vi "Set_Traverse_Position.vi"(3 "Last Part of Move?":bool=TRUE, 4 "Currently on Point":i32=11, 5 "Simulate/Run":T3, 6 "Traverse line":T4 {"Carrier_2 Q (l/min)" format="%#.2f"; "Row Duration (mins)" format="%#.1f"; "Row No" min=0; "Trace Gas Concentration (%)" min=0.0 format="%#_4f"; "Carrier_1 Q (l/min)" format="%#.4f"; "Start X" format="%#.2f"; "Start Y" format="%#.2f"; "Start Z" format="%#.2f"; "End X" format="%#.2f"; "End Y" format="%#.2f"; "End Z" format="%#.2f"; "Tunnel Speed" format="%#.2f"; "Averaging time (mins)" min=0.0 format="%#.2f"}) -> (0 "Status Cluster":T1)   [LabVIEW 2021]
uses:
  Traverse_cluster.ctl
  Spacing.ctl
  Controls/Multi_run_mode.ctl
  Controls/User_Specific_mode.ctl
  Status_Cluster.ctl
  Multi_Run_Status.ctl
  Controls/Home.ctl
  Globals/Extra_Commands_Global.vi
  Globals/Dynamic_call_global.ph.vi
  Globals/Constants_global.vi
panel:
  # "X           Y          Z"
  # "Start"
  # "End"
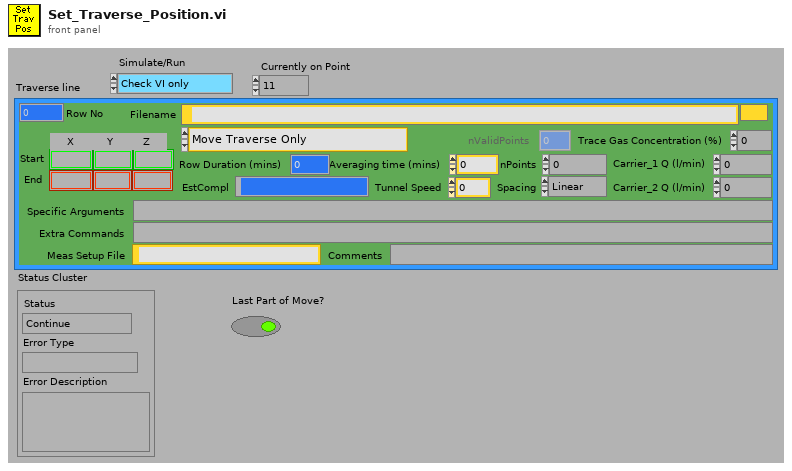
[diagram p1: front panel]
types:
  T1 = typedef "Status_Cluster.ctl" = cluster{"Status":T2, "Error Type":string, "Error Description":string}
  T2 = typedef "Multi_Run_Status.ctl" = enum16{"Continue", "Continue with Error", "Jump to Next Point", "Jump to Next Row", "Jump To Fall Back", "Terminate Run"}
  T3 = typedef "User_Specific_mode.ctl" = enum16{"Check VI only", "Run VI"}
  T4 = typedef "Traverse_cluster.ctl" = cluster{"Start X":sgl, "Start Y":sgl, "Start Z":sgl, "End X":sgl, "End Y":sgl, "End Z":sgl, "nPoints":i32, "Spacing":T5, "Filename":path, "Tunnel Speed":dbl, "Averaging time (mins)":dbl, "Extra Commands":string, "Carrier_1 Q (l/min)":dbl, "Carrier_2 Q (l/min)":dbl, "Trace Gas Concentration (%)":dbl, "Specific Arguments":string, "Comments":string, "Row No":i32, "Row Type Selector":T6, "EstCompl":string, "Row Duration (mins)":dbl, "nValidPoints":i32, "Meas Setup File":string}
  T5 = typedef "Spacing.ctl" = enum16{"Linear", "Log", "Gauss", "Specified", "N/A"}
  T6 = typedef "Multi_run_mode.ctl" = enum16{"Move Traverse Only", "Set Tunnel Speed Only", "Set Source Only", "Set Measurement Conditions", "Single Measurement", "Vertical Profile", "Lateral Profile", "Longitudinal Profile", "Multi-Axis Profile", "Explore Volume", "Auto Calibrate", "Meas Fast FID Bkgnd", "Check Beam Power", "Scanning Valve Measurement", "Run VI Named:", "Set ADAM Ch", "Wait (minutes)", "Send Message", "Synchronize With:", "Fall Back to this Row", "Turn Off Row Repeating", "Traverse 3D Volume", "Blank Row", "Jump to Fall Back Row"}
  T7 = typedef "Home.ctl" = enum16{"Don't Home", "Home  +X", "Home  -X", "Home  +Y", "Home  -Y", "Home  +Z", "Home  -Z"}
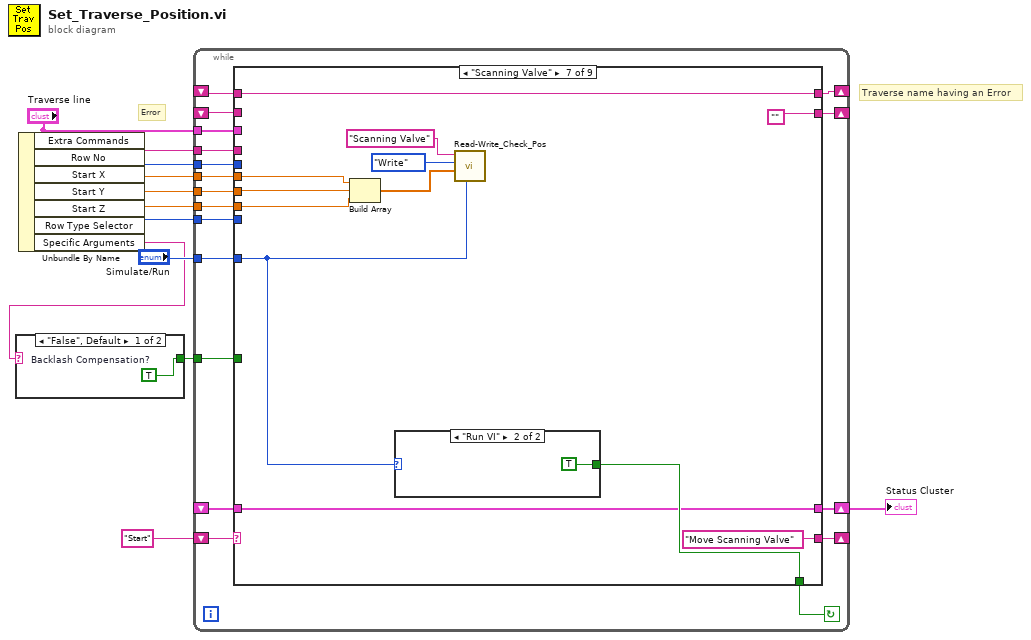
[diagram p0: block diagram]
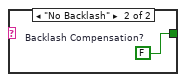
[diagram p2: hidden frame]
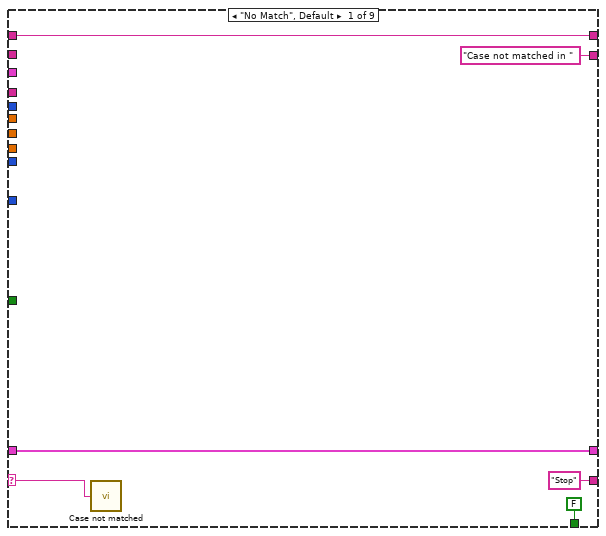
[diagram p3: hidden frame]
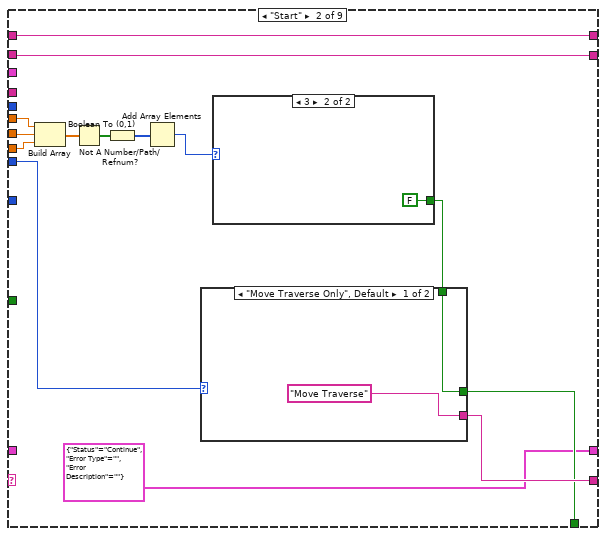
[diagram p4: hidden frame]
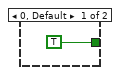
[diagram p5: hidden frame]
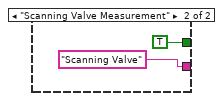
[diagram p6: hidden frame]
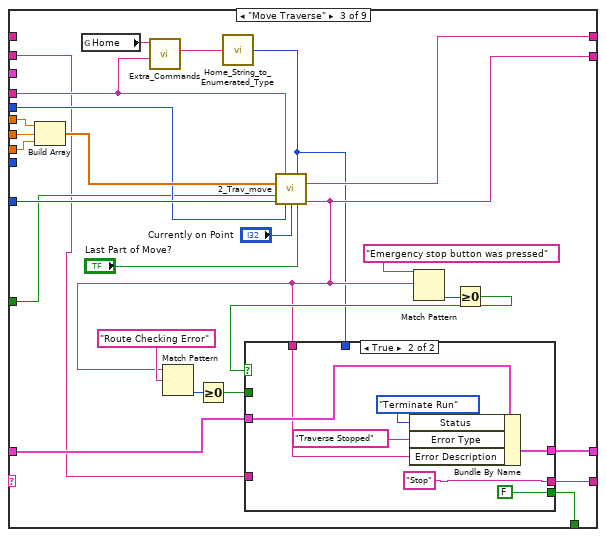
[diagram p7: hidden frame]
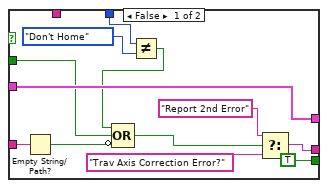
[diagram p8: hidden frame]
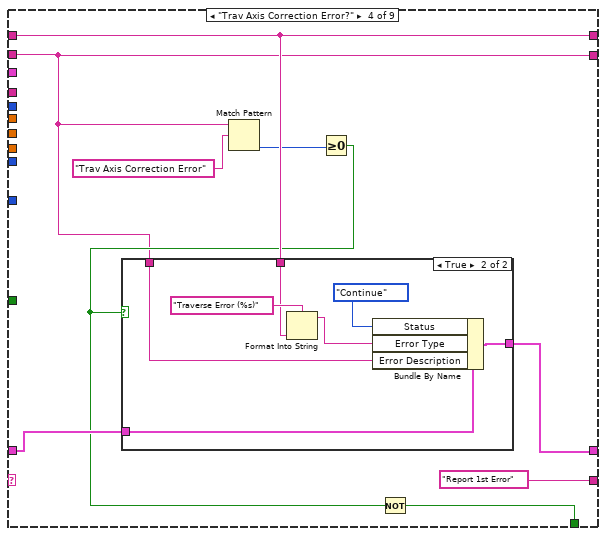
[diagram p9: hidden frame]
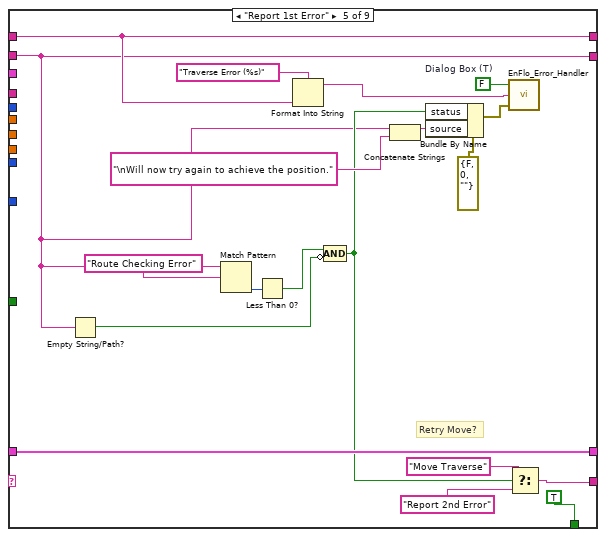
[diagram p11: hidden frame]
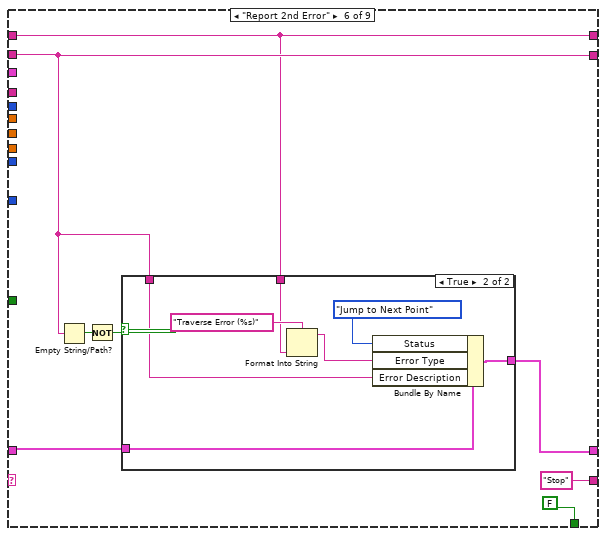
[diagram p12: hidden frame]
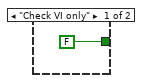
[diagram p14: hidden frame]
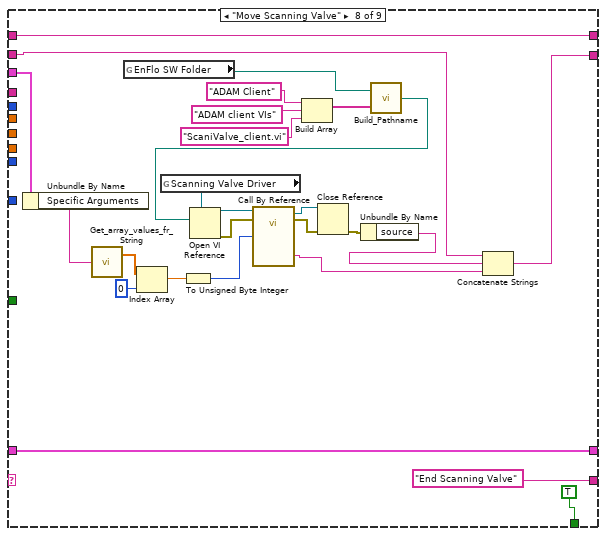
[diagram p15: hidden frame]
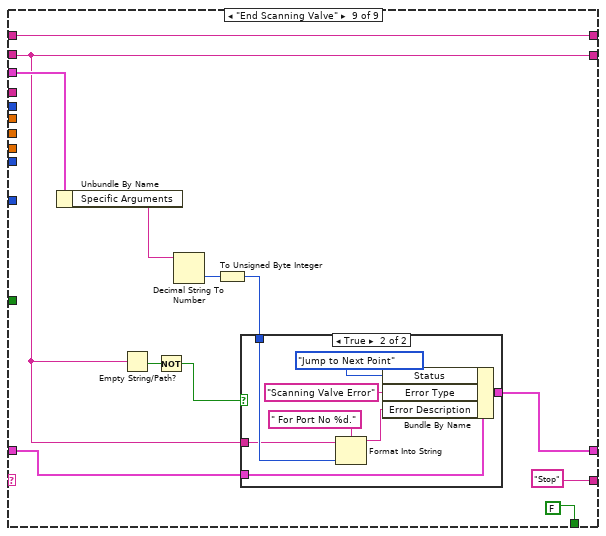
[diagram p16: hidden frame]
diagram:
  # "Traverse name having an Error"
  # "Error"
  n1 = Unbundle By Name("Traverse line") -> ("Extra Commands"=w11:string, "Row No"=w10:i32, "Start X"=w8:sgl, "Start Y"=w12:sgl, "Start Z"=w7:sgl, "Row Type Selector"=w9:T6, "Specific Arguments"=w3:string)
  n2 = case shown="\"False\", Default" w3 {
    tunnel: [w13 w14] -> w2
    frame "False", Default {
      w13 = TRUE  # Backlash Compensation?
    }
    frame "No Backlash" {
      w14 = FALSE  # Backlash Compensation?
    }
  }
  n3 = while {
    shift-left: _ -> [w19]
    shift-right: [w20] -> _
    shift-left: _ -> [w21]
    shift-right: [w22] -> w4
    tunnel: "Traverse line" -> [w23]
    tunnel: "Simulate/Run" -> [w24]
    tunnel: w7 -> [w25]
    tunnel: w12 -> [w26]
    tunnel: w8 -> [w27]
    tunnel: w9 -> [w30]
    shift-left: "Start" -> [w15]
    shift-right: [w28] -> _
    tunnel: w10 -> [w31]
    tunnel: w11 -> [w32]
    tunnel: w2 -> [w18]
    shift-right: [w17] -> _
    shift-left: _ -> [w16]
    stop <- w29 continue-if-true
    n4 = case shown="\"Scanning Valve\"" w15 {
      selector: w15 -> [w33 _ _ _ _ _ _ _ _]
      tunnel: w32 -> [_ _ w64 _ _ _ _ _ _]
      tunnel: w31 -> [_ _ w77 _ _ _ _ _ _]
      tunnel: w30 -> [_ w52 _ _ _ _ _ _ _]
      tunnel: [FALSE w50 w71 w106 TRUE FALSE w167 TRUE FALSE] -> w29
      tunnel: ["Stop" w51 w78 "Report 1st Error" w128 "Stop" "Move Scanning Valve" "End Scanning Valve" "Stop"] -> w28
      tunnel: w27 -> [_ w45 w83 _ _ _ w161 _ _]
      tunnel: w26 -> [_ w46 w82 _ _ _ w160 _ _]
      tunnel: w25 -> [_ w47 w81 _ _ _ w159 _ _]
      tunnel: w24 -> [_ _ w79 _ _ _ w156 _ _]
      tunnel: w23 -> [_ _ _ _ _ _ _ w189 w206]
      tunnel: [w36 T1 {"Status"=enum."Continue", "Error Type"="", "Error Description"=""} ("Status Cluster") w73 w111 w134 w146 w166 w180 w203] -> w22
      tunnel: w21 -> [w36 _ w72 w112 w134 w147 w166 w180 w204]
      tunnel: ["Case not matched in " ("Error String") w48 w69 w105 w121 w143 "" w173 w198] -> w20
      tunnel: w19 -> [_ w48 w63 w105 w121 w143 _ w172 w198]
      tunnel: w18 -> [_ _ w66 _ _ _ _ _ _]
      tunnel: [w38 w44 w65 w110 w124 w141 w158 w171 w197] -> w17
      tunnel: w16 -> [w38 w44 _ w110 w124 w141 w158 w171 w197]
      frame "No Match", Default {
        n5 = call "Case not matched.vi"("Case Name not Matched"=w33) -> ()
      }
      frame "Start" {
        n6 = Build Array(w45, w46, w47) -> (w41:sgl[])
        n7 = Not A Number/Path/Refnum?(number/path/refnum=w41) -> (NaN/Path/Refnum?=w42:bool[])
        n8 = Boolean To (0,1)(Boolean=w42) -> (0, 1=w43:i16[])
        n9 = Add Array Elements(numeric array=w43) -> (sum=w40:i16)
        n10 = case shown="3" w40 {
          tunnel: [TRUE FALSE] -> w39
          frame 0, Default {
          }
          frame 3 {
          }
        }
        n11 = case shown="\"Move Traverse Only\", Default" w52 {
          tunnel: ["Move Traverse" "Scanning Valve"] -> w51
          tunnel: [w56 TRUE] -> w50
          tunnel: w39 -> [w56 _]
          frame "Move Traverse Only", Default {
          }
          frame "Scanning Valve Measurement" {
          }
        }
      }
      frame "Move Traverse" {
        n12 = Build Array(w83, w82, w81) -> (w80:sgl[])
        n13 = global read "Extra_Commands_Global.vi" "Home"() -> (w62:string)
        n14 = call "Extra_Commands.vi"("String to Search"=w64, "Command"=w62) -> ("String Value"=w61:string)  [unwired: 1 in, 4 out]
        n15 = call "Home_String_to_Enumerated_Type.vi"("String"=w61) -> ("Home"=w60:T7)
        n16 = call "2_Trav_move.vi"("Extra Command String"=w64, "Home Z"=w60, "New Position"=w80, "Backlash Compensation?"=w66, "Simulate/Run"=w79, "Row Number"=w77, "Currently on Point"="Currently on Point", "Last Part of Move?"="Last Part of Move?") -> ("Error from Traverse named"=w65:string, "Error String"=w69:string)  [unwired: 5 in, 1 out]
        n17 = Match Pattern(string=w69, regular expression="Route Checking Error") -> (offset past match=w68:i32)  [unwired: 4 out]
        n18 = Greater Or Equal To 0?(x=w68) -> (x >= 0?=w67:bool)
        n19 = Match Pattern(string=w69, regular expression="Emergency stop button was pressed") -> (offset past match=w75:i32)  [unwired: 4 out]
        n20 = Greater Or Equal To 0?(x=w75) -> (x >= 0?=w74:bool)
        n21 = case shown="True" w74 {
          tunnel: [w96 "Stop"] -> w78
          tunnel: w63 -> [w95 _]
          tunnel: [w94 w100] -> w73
          tunnel: w72 -> [w94 w101]
          tunnel: w69 -> [_ w99]
          tunnel: [TRUE FALSE] -> w71
          tunnel: w67 -> [w92 _]
          tunnel: w60 -> [w89 _]
          frame False {
            n22 = Empty String/Path?(string/path=w95) -> (empty?=w90:bool)
            n23 = Not Equal?(x=w89, y=Home."Don't Home" ("Home")) -> (x != y?=w87:bool)
            n24 = Compound Arithmetic op=OR(w87, w92, invert w90) -> (w91:bool)
            n25 = Select(t="Report 2nd Error", s=w91, f="Trav Axis Correction Error?") -> (s? t:f=w96:string)
          }
          frame True {
            n26 = Bundle By Name(cluster=w101, "Status"=Multi_Run_Status."Terminate Run", "Error Type"="Traverse Stopped" ("t"), "Error Description"=w99) -> (w100:T1)
          }
        }
      }
      frame "Trav Axis Correction Error?" {
        n27 = Match Pattern(string=w105, regular expression="Trav Axis Correction Error" ("string")) -> (offset past match=w109:i32)  [unwired: 4 out]
        n28 = Greater Or Equal To 0?(x=w109) -> (x >= 0?=w107:bool)
        n29 = case shown="True" w107 {
          tunnel: w112 -> [w113 w120]
          tunnel: [w113 w118] -> w111
          tunnel: w105 -> [_ w117]
          tunnel: w110 -> [_ w114]
          frame False {
          }
          frame True {
            n30 = Format Into String(format string="Traverse Error (%s)" ("t"), w114) -> (resulting string=w115:string)  [unwired: 2 in, 1 out]
            n31 = Bundle By Name(cluster=w120, "Status"=Multi_Run_Status."Continue", "Error Type"=w115, "Error Description"=w117) -> (w118:T1)
          }
        }
        n32 = Not(x=w107) -> (.not. x?=w106:bool)
      }
      frame "Report 1st Error" {
        w137 = FALSE  # Dialog Box (T)
        # "Retry Move?"
        n33 = Empty String/Path?(string/path=w121) -> (empty?=w127:bool)
        n34 = Match Pattern(string=w121, regular expression="Route Checking Error" ("String to match")) -> (offset past match=w131:i32)  [unwired: 4 out]
        n35 = Less Than 0?(x=w131) -> (x < 0?=w130:bool)
        n36 = Format Into String(format string="Traverse Error (%s)" ("t"), w124) -> (resulting string=w125:string)  [unwired: 2 in, 1 out]
        n37 = Compound Arithmetic op=AND(w130, invert w127) -> (w129:bool)
        n38 = Concatenate Strings(w121, "\nWill now try again to achieve the position." ("Substring")) -> (w136:string)
        n39 = Bundle By Name(cluster=errorcluster {"status"=FALSE, "code"=0, "source"=""} ("error in (no error)"), "status"=w129, "source"=w136) -> (w138:errorcluster)
        n40 = call "EnFlo_Error_Handler.vi"("error in (no error)"=w138, "Error Type"=w125, "Dialog Box (F)"=w137) -> ()  [unwired: 3 out]
        n41 = Select(t="Move Traverse", s=w129, f="Report 2nd Error") -> (s? t:f=w128:string)
      }
      frame "Report 2nd Error" {
        n42 = Empty String/Path?(string/path=w143) -> (empty?=w144:bool)
        n43 = Not(x=w144) -> (.not. x?=w142:bool)
        n44 = case shown="True" w142 {
          tunnel: w147 -> [w148 w155]
          tunnel: [w148 w153] -> w146
          tunnel: w143 -> [_ w152]
          tunnel: w141 -> [_ w149]
          frame False {
          }
          frame True {
            n45 = Format Into String(format string="Traverse Error (%s)" ("t"), w149) -> (resulting string=w150:string)  [unwired: 2 in, 1 out]
            n46 = Bundle By Name(cluster=w155, "Status"=Multi_Run_Status."Jump to Next Point", "Error Type"=w150, "Error Description"=w152) -> (w153:T1)
          }
        }
      }
      frame "Scanning Valve" {
        n47 = Build Array(w161, w160, w159) -> (w164:sgl[])
        n48 = case shown="\"Run VI\"" w156 {
          tunnel: [FALSE TRUE] -> w167
          frame "Check VI only" {
          }
          frame "Run VI" {
          }
        }
        n49 = call "Read-Write_Check_Pos.vi"("Simulate/Run"=w156, "Position input"=w164, "Mode"=enum16{"Read", "Write"}."Write", "Traverse Name"="Scanning Valve") -> ()  [unwired: 3 in, 3 out]
      }
      frame "Move Scanning Valve" {
        n50 = Unbundle By Name(w189) -> ("Specific Arguments"=w177:string)
        n51 = call "Get_array_values_fr_String.vi"("String Value"=w177) -> ("Numeric Array"=w179:dbl[])  [unwired: 1 out]
        n52 = global read "Constants_global.vi" "EnFlo SW Folder"() -> (w183:path)
        n53 = Index Array(array=w179, index=0) -> (element=w176:dbl)
        n54 = global read "Dynamic_call_global.ph.vi" "Scanning Valve Driver"() -> (w190:refnum<vi>)
        n55 = To Unsigned Byte Integer(number=w176) -> (unsigned 8bit integer=w188:u8)
        n56 = Build Array("ADAM Client", "ADAM client VIs", "ScaniValve_client.vi") -> (w184:string[])
        n57 = call "Build_Pathname.vi"("PathElements"=w184, "PathnameIn"=w183) -> ("AppendedPath"=w182:path)
        n58 = Open VI Reference(type specifier VI Refnum (for type only)=w190, vi path=w182) -> (vi reference=w191:refnum<vi>, error out=w192:errorcluster)  [unwired: 2 in, 2 out]
        n59 = call-by-ref "?"(reference=w191, error in=w192, "Port Number"=w188) -> (reference out=w194:refnum<vi>, error out=w193:errorcluster, "Error String"=w174:string)  [unwired: 2 out]
        n60 = Close Reference(reference=w194, error in (no error)=w193) -> (error out=w195:errorcluster)
        n61 = Unbundle By Name(w195) -> ("source"=w175:string)
        n62 = Concatenate Strings(w172, w175, w174) -> (w173:string)
      }
      frame "End Scanning Valve" {
        n63 = Unbundle By Name(w206) -> ("Specific Arguments"=w207:string)
        n64 = Empty String/Path?(string/path=w198) -> (empty?=w200:bool)
        n65 = Not(x=w200) -> (.not. x?=w199:bool)
        n66 = Decimal String To Number(string=w207) -> (number=w205:i32)  [unwired: 3 out]
        n67 = To Unsigned Byte Integer(number=w205) -> (unsigned 8bit integer=w202:u8)
        n68 = case shown="True" w199 {
          tunnel: w204 -> [w208 w216]
          tunnel: [w208 w213] -> w203
          tunnel: w202 -> [_ w211]
          tunnel: w198 -> [_ w209]
          frame False {
          }
          frame True {
            n69 = Format Into String(format string=" For Port No %d." ("Format String"), initial string=w209, w211) -> (resulting string=w210:string)  [unwired: 1 in, 1 out]
            n70 = Bundle By Name(cluster=w216, "Status"=Multi_Run_Status."Jump to Next Point", "Error Type"="Scanning Valve Error" ("t"), "Error Description"=w210) -> (w213:T1)
          }
        }
      }
    }
  }
  "Status Cluster" <- w4
